vi "HIDinRealTime1.vi"() -> ()   [LabVIEW 2015]
panel:
  out "Hold Time":i64
  out "Pressed Sequence":string[](array[string])
  in  "stop":bool
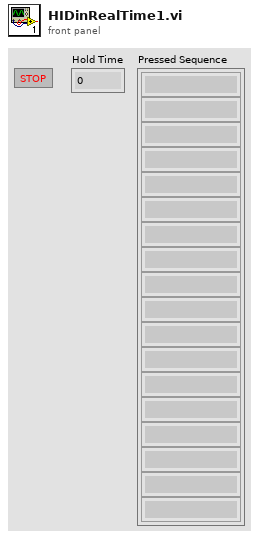
[diagram p1: front panel]
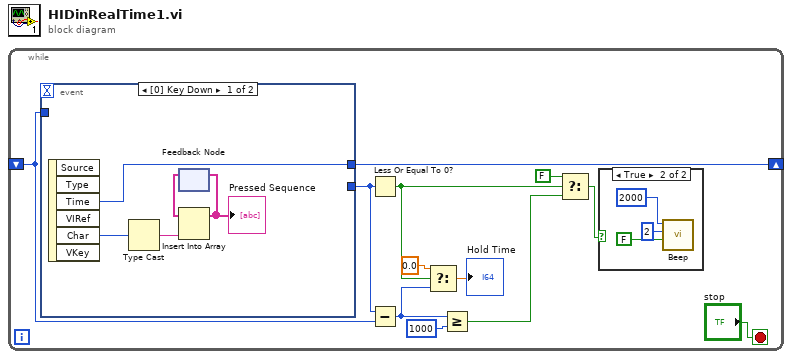
[diagram p0: block diagram]
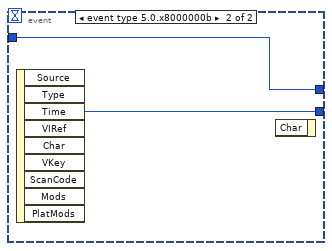
[diagram p3: hidden frame]
diagram:
  n1 = while {
    shift-right: [w10] -> _
    shift-left: _ -> [w9]
    stop <- "stop" stop-if-true
    n2 = event shown="[0] Key Down" {
      selector: _ -> [_ _]
      dyn-events: _ -> [_ _]
      timeout: _ -> [_ _]
      tunnel: [w16 w21] -> w10
      tunnel: [_ w22] -> w8
      tunnel: w9 -> [_ w21]
      event Key Down {
        n3 = event-data() -> ("Time"=w16:u32, "Char"=w17:i16)  [unwired: 1 in, 4 out]
        n4 = Type Cast(x=w17) -> (*(type *) &x=w18:string)  [unwired: 1 in]
        n5 = feedback #1() -> (w20:string[])  [unwired: 1 in]
        n6 = Insert Into Array(array=w20, new element=w18) -> (w19:string[])  [unwired: 1 in]
        "Pressed Sequence" <- w19
        n7 = feedback-in #1(w19) -> ()
      }
      event event type 5.0.x8000000b {
        n8 = event-data() -> ("Time"=w22:u32)  [unwired: 1 in, 8 out]
        n9 = event-data() -> ()  [unwired: 2 in, 1 out]
      }
    }
    n10 = Less Or Equal To 0?(x=w8) -> (x <= 0?=w5:bool)
    n11 = Subtract(x=w8, y=w9) -> (x-y=w3:u32)
    n12 = Select(t=0.0, s=w5, f=w3) -> (s? t:f=→"Hold Time":dbl)
    n13 = Greater Or Equal?(x=w3, y=u32 1000) -> (x >= y?=w1:bool)
    n14 = Select(t=FALSE, s=w5, f=w1) -> (s? t:f=w6:bool)
    n15 = case shown="True" w6 {
      frame False {
      }
      frame True {
        n16 = call <vilib>:"Beep.vi"("use system alert? (T)"=FALSE, "duration (msec)"=u32 2, "frequency (Hz)"=u32 2000) -> ()  [unwired: 9 in]
      }
    }
  }
